vi "Vector Addition.vi"(8 "error in (no error)":errorcluster) -> (0 "error out":errorcluster)   [LabVIEW 2023]
uses:
  <vilib>/addons/_JKI Toolkits/Caraya/classes/Assert/Assert True.vi
  <vilib>/addons/_JKI Toolkits/Caraya/classes/Test/Test.lvclass
  <vilib>/addons/_JKI Toolkits/Caraya/classes/Assert/Assert.lvclass
panel:
  # "Connector Pane"
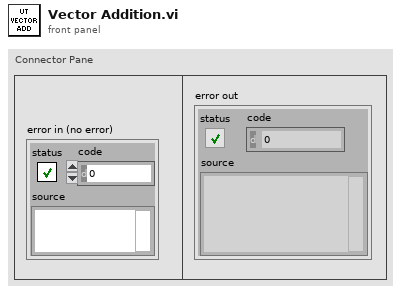
[diagram p1: front panel]
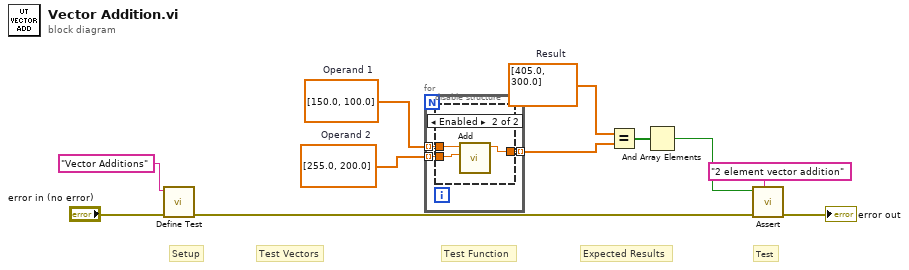
[diagram p0: block diagram]
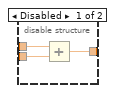
[diagram p2: hidden frame]
diagram:
  w3 = dbl[] [405.0, 300.0]  # Result
  w6 = dbl[] [255.0, 200.0]  # Operand 2
  w7 = dbl[] [150.0, 100.0]  # Operand 1
  # "Test Function"
  # "Expected Results"
  # "Test Vectors"
  # "Test"
  # "Setup"
  n1 = call <vilib>:"Define Test.vi"("error in (no error)"="error in (no error)", "Label (VI Title)"="Vector Additions") -> ("error out"=w8:errorcluster)  [unwired: 9 in]
  n2 = for {
    tunnel: w7 -> [w14] mode=indexing
    tunnel: w6 -> [w13] mode=indexing
    tunnel: [w12] -> w5 mode=indexing
    n3 = disable-structure shown="Enabled" {
      disable-tunnel: w14 -> [w17 w20]
      disable-tunnel: w13 -> [w16 w19]
      disable-tunnel: [w15 w18] -> w12
      frame Disabled {
        n4 = Add(x=w17, y=w16) -> (x+y=w15:dbl)
      }
      frame Enabled {
        n5 = call "Add.vi"("Operand 2"=w19, "Operand 1"=w20) -> ("Numeric"=w18:dbl)  [unwired: 9 in]
      }
    }
  }
  n6 = Equal?(x=w3, y=w5) -> (x = y?=w4:bool[])
  n7 = And Array Elements(Boolean array=w4) -> (logical AND=w1:bool)
  n8 = call-poly <vilib>:"Assert.vi"("Label"="2 element vector addition" ("Label (VI Title)"), "error in (no error)"=w8, "True?"=w1) -> ("error out"=→"error out":errorcluster)  [unwired: 8 in]
